vi "MGCC_StaEst_main_HTB.vi"() -> ()   [LabVIEW 2016]
doc: "----------------------------------------------------------------------------------------------------------------\nCopyright <2019> <The University of Tennessee at Knoxville and the University of Tennessee Research Foundation>\nThis software is released under BSD-3 \nhttps://opensource.org/licenses/BSD-3-Clause \nAdditional license options available at https://utrf.tennessee.edu/industry/sample-agreements/\n----------------------------------------------------------------------------------------------------------------\n\n\nThis VI is designed for the state estimation function block. The current version is designed for IEEE13node system. The advanced model will be available in the latest version. There is no input for this VI. Bascially, the input right now comes from the cvs in IEEE13 folder."
uses:
  Finite State Machine/Sub-VIs/MGCC_FntStaMach_gobal.vi
  Model Management/Global_MdlMgmt.vi
panel:
  out "st_MGCC_StaEst_Input":T1
  in  "vbase":dbl=6928.4
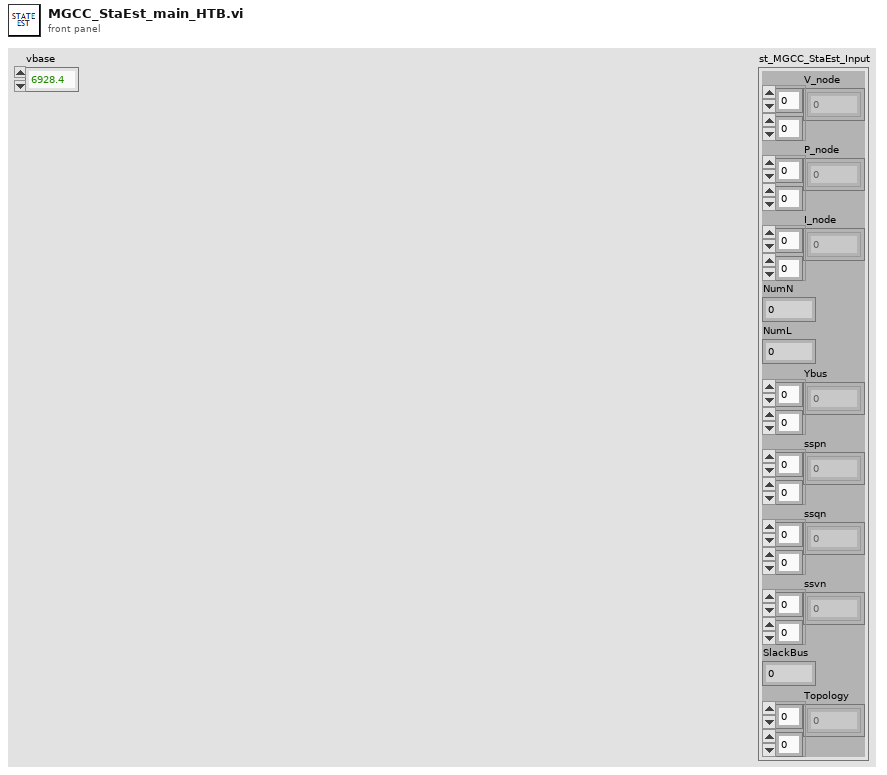
[diagram p1: front panel]
types:
  T1 = cluster{"V_node":cdb[][], "P_node":cdb[][], "I_node":cdb[][], "NumN":dbl, "NumL":dbl, "Ybus":cdb[][], "sspn":dbl[][], "ssqn":dbl[][], "ssvn":dbl[][], "SlackBus":dbl, "Topology":dbl[][]}
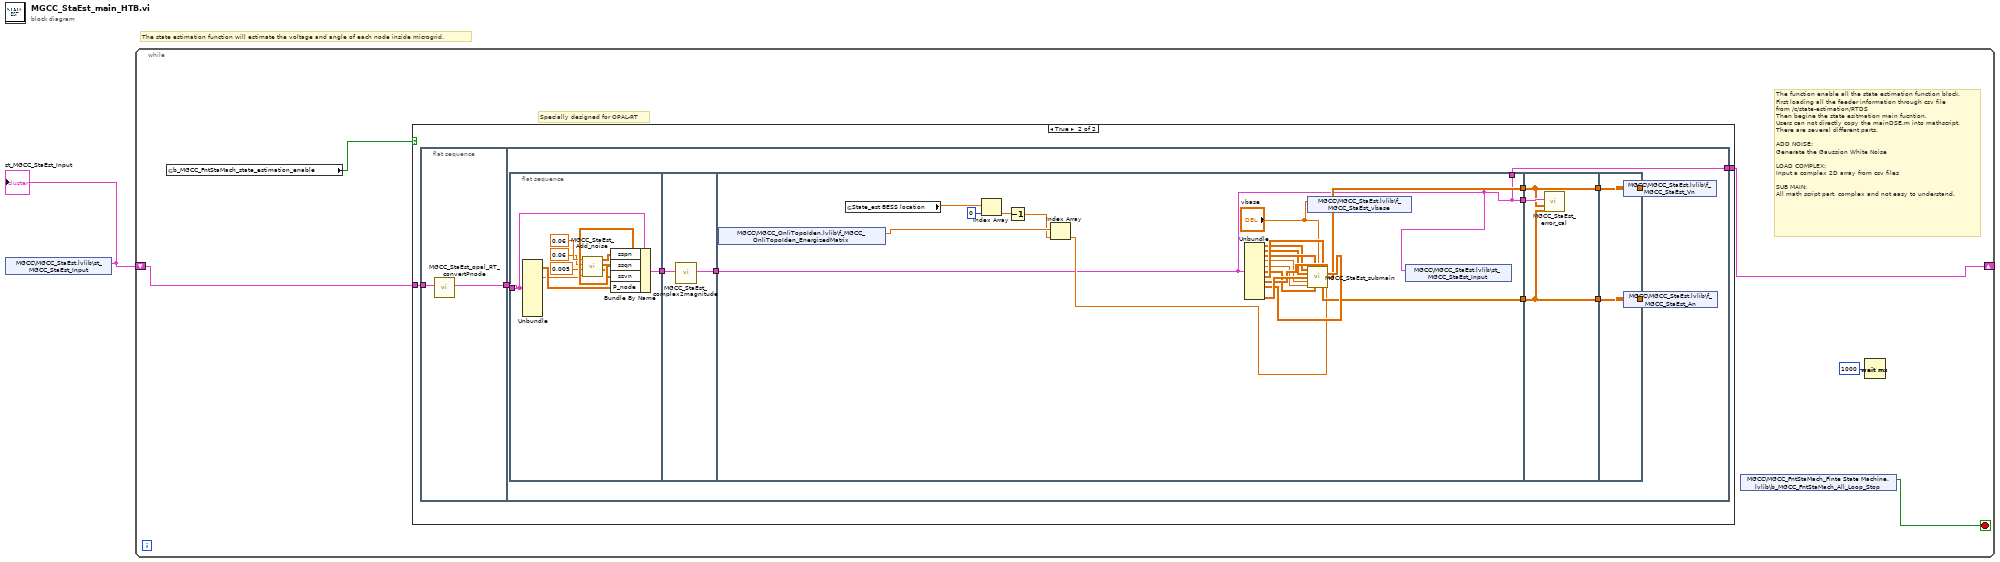
[diagram p0: block diagram]
diagram:
  # "The state estimation function will estimate the voltage and angle of each node inside microgrid."
  n1 = shared-variable "MGCC\\MGCC_StaEst.lvlib\\st_MGCC_StaEst_Input"() -> (w1:T1)  [unwired: 1 in, 1 out]
  "st_MGCC_StaEst_Input" <- w1
  n2 = while {
    shift-right: [w3] -> _
    shift-left: w1 -> [w4]
    stop <- w6 stop-if-true
    # "Specially designed for OPAL-RT"
    # "The function enable all the state estimation function block.\nFirst loading all the feeder information through csv file\nfrom /c/state-estimation/RTDS\nThen begine the state esitmation main fucntion.\nUsers can not directly copy the mainDSE.m into mathscript.\nThere are several different parts.\n\nADD NOISE:\nGenerate the Gaussion White Noise\n\nLOAD COMPLEX:\nInput a complex 2D array from csv files\n\nSUB MAIN:\nAll math script part, complex and not easy to understand."
    n3 = global read "MGCC_FntStaMach_gobal.vi" "b_MGCC_FntStaMach_state_estimation_enable"() -> (w2:bool)
    n4 = case shown="True" w2 {
      tunnel: w4 -> [w7 w9]
      tunnel: [w7 w8] -> w3
      frame False {
      }
      frame True {
        n5 = flat-sequence {
          tunnel: [w12] -> w10
          tunnel: w9 -> [w11]
          tunnel: w10 -> [w17]
          tunnel: [w13] -> w8
          frame #0 {
            n6 = call "MGCC_StaEst_opal_RT_convertPnode.vi"("cluster"=w11) -> ("P_node"=w12:T1)  [unwired: 10 in]
          }
          frame #1 {
            n7 = flat-sequence {
              tunnel: w17 -> [w32]
              tunnel: [w31] -> w16
              tunnel: w16 -> [w34]
              tunnel: [w35] -> w15
              tunnel: [w45] -> w23
              tunnel: [w44] -> w22
              tunnel: w15 -> [w38]
              tunnel: [w38] -> w14
              tunnel: [w38] -> w13
              tunnel: [w57] -> w21
              tunnel: w23 -> [w57]
              tunnel: [w56] -> w20
              tunnel: w22 -> [w56]
              tunnel: w14 -> [w58]
              tunnel: [w60] -> w19
              tunnel: [w59] -> w18
              tunnel: w21 -> [w60]
              tunnel: w20 -> [w59]
              frame #0 {
                n8 = Unbundle(w32) -> ("P_node"=w33:cdb[][], "NumN"=w24:dbl)  [unwired: 9 out]
                n9 = call "MGCC_StaEst_Add_noise.vi"("spn"=0.06, "sqn"=0.06, "svn"=0.005, "Node"=w24) -> ("sspn"=w30:dbl[][], "ssvn"=w29:dbl[][], "ssqn"=w28:dbl[][])  [unwired: 2 in]
                n10 = Bundle By Name(cluster=w32, "sspn"=w30, "ssqn"=w29, "ssvn"=w28, "P_node"=w33) -> (w31:T1)
              }
              frame #1 {
                n11 = call "MGCC_StaEst_complex2magnitude.vi"("st_MGCC_StaEst_Input"=w34) -> ("output cluster"=w35:T1)  [unwired: 10 in]
              }
              frame #2 {
                n12 = shared-variable "MGCC\\MGCC_OnliTopoIden.lvlib\\f_MGCC_OnliTopoIden_EnergizedMatrix"() -> (w40:dbl[])  [unwired: 1 in, 1 out]
                n13 = global read "Global_MdlMgmt.vi" "State_est BESS location"() -> (w42:dbl[])
                n14 = Index Array(array=w42, index=0) -> (element=w37:dbl)
                n15 = Decrement(x=w37) -> (x-1=w36:dbl)
                n16 = Index Array(array=w40, index=w36) -> (element=w39:dbl)
                n17 = Unbundle(w38) -> ("V_node"=w47:cdb[][], "P_node"=w43:cdb[][], "I_node"=w48:cdb[][], "NumN"=w49:dbl, "NumL"=w50:dbl, "Ybus"=w51:cdb[][], "sspn"=w52:dbl[][], "ssqn"=w53:dbl[][], "ssvn"=w54:dbl[][], "Topology"=w55:dbl[][])  [unwired: 1 out]
                n18 = shared-variable "MGCC\\MGCC_StaEst.lvlib\\f_MGCC_StaEst_vbase"("vbase") -> ()  [unwired: 1 in, 1 out]
                n19 = call "MGCC_StaEst_submain.vi"("V_node"=w47, "I_node"=w48, "vbase"="vbase", "sspn"=w52, "ssqn"=w53, "P_node"=w43, "ssvn"=w54, "Topology"=w55, "NumN"=w49, "NumL"=w50, "Ybus"=w51, "interrupt"=w39) -> ("VN"=w45:dbl[][], "AN"=w44:dbl[][])  [unwired: 1 in, 1 out]
                n20 = shared-variable "MGCC\\MGCC_StaEst.lvlib\\st_MGCC_StaEst_Input"(w38) -> ()  [unwired: 1 in, 1 out]
              }
              frame #3 {
                n21 = call "MGCC_StaEst_error_cal.vi"("f_MGCC_StaEst_An"=w56, "f_MGCC_StaEst_Vn"=w57, "cluster"=w58) -> ()  [unwired: 9 in]
              }
              frame #4 {
              }
            }
            n22 = shared-variable "MGCC\\MGCC_StaEst.lvlib\\f_MGCC_StaEst_Vn"(w19) -> ()  [unwired: 1 in, 1 out]
            n23 = shared-variable "MGCC\\MGCC_StaEst.lvlib\\f_MGCC_StaEst_An"(w18) -> ()  [unwired: 1 in, 1 out]
          }
        }
      }
    }
    n24 = shared-variable "MGCC\\MGCC_FntStaMach_Finte State Machine.lvlib\\b_MGCC_FntStaMach_All_Loop_Stop"() -> (w6:bool)  [unwired: 1 in, 1 out]
    n25 = Wait (ms)(milliseconds to wait=u32 1000) -> ()  [unwired: 1 out]
  }
